vi "single_color_3D_continuous_scan_with_delay_and_ETL_control.vi"() -> ()   [LabVIEW 2017]
uses:
  <vilib>/DAQmx/write.llb/DAQmx Write (Analog DBL 1Chan 1Samp).vi
  <vilib>/DAQmx/write.llb/DAQmx Write (Analog 1D DBL NChan 1Samp).vi
  <vilib>/DAQmx/write.llb/DAQmx Write (Analog 2D DBL NChan NSamp).vi
  <vilib>/DAQmx/create/channels.llb/DAQmx Create Channel (AO-Voltage-Basic).vi
  <vilib>/DAQmx/miscellaneous.llb/DAQmx Fill In Error Info.vi
  <vilib>/Utility/file.llb/Read Delimited Spreadsheet (DBL).vi
  <vilib>/measure/mascope.llb/Transition Measurements 1 chan.vi
  <vilib>/DAQmx/configure/timing.llb/DAQmx Timing (Sample Clock).vi
  <vilib>/DAQmx/configure/trigger.llb/DAQmx Start Trigger (Digital Edge).vi
  <vilib>/DAQmx/configure/trigger.llb/DAQmx Start Trigger (None).vi
  <vilib>/measure/NI_MAPro.lvlib
panel:
  in  "Listbox":i32(listbox)=3
  in  "ETL3 (v)":dbl(slide) scale=-10.0..10.0
  out "mirx raw 2":dbl[](array[numeric])
  out "Delay":dbl
  out "Sampling rate":i32
  out "ETL3":waveform(dbl)(graph)
  out "mirror y":waveform(dbl)(graph)
  out "mirror x":waveform(dbl)(graph)
  out "Laser":waveform(dbl)(graph)
  out "camera":waveform(dbl)(graph)
  out "mirx transition duration":dbl
  out "etl3 timing array":dbl[](array[numeric])
  out "mirror y timing array":dbl[](array[numeric])
  out "mirror x timing array":dbl[](array[numeric])
  out "Laser timing array":dbl[](array[numeric])
  out "camera timing array":dbl[](array[numeric])
  out "etl raw":dbl[](array[numeric])
  out "miry raw":dbl[](array[numeric])
  out "mirx raw":dbl[](array[numeric])
  out "Laser Intensity":dbl
  out "Off Time":dbl
  out "On Time":dbl
  out "Number of slices":dbl
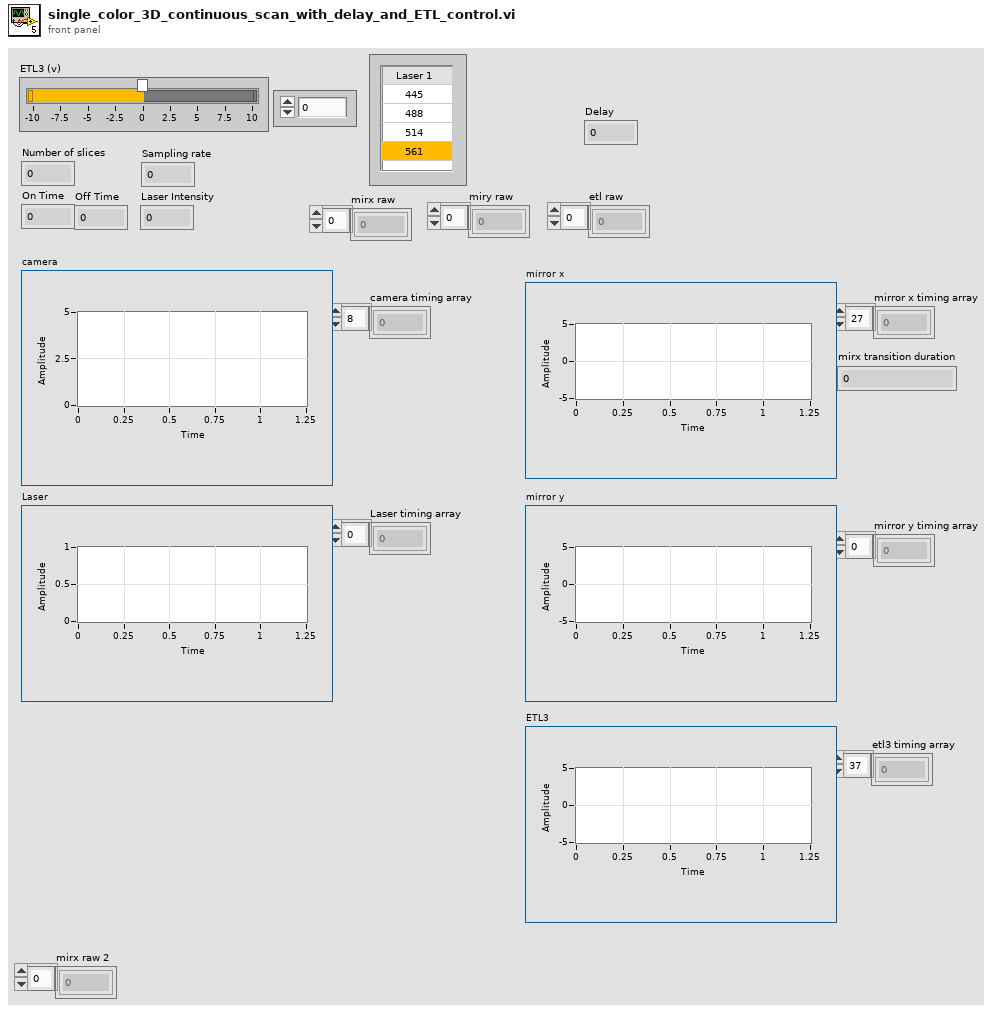
[diagram p1: front panel]
types:
  T1 = enum32{"Invalid", "Standard", "Closed", "Hidden", "Minimized", "Maximized"}
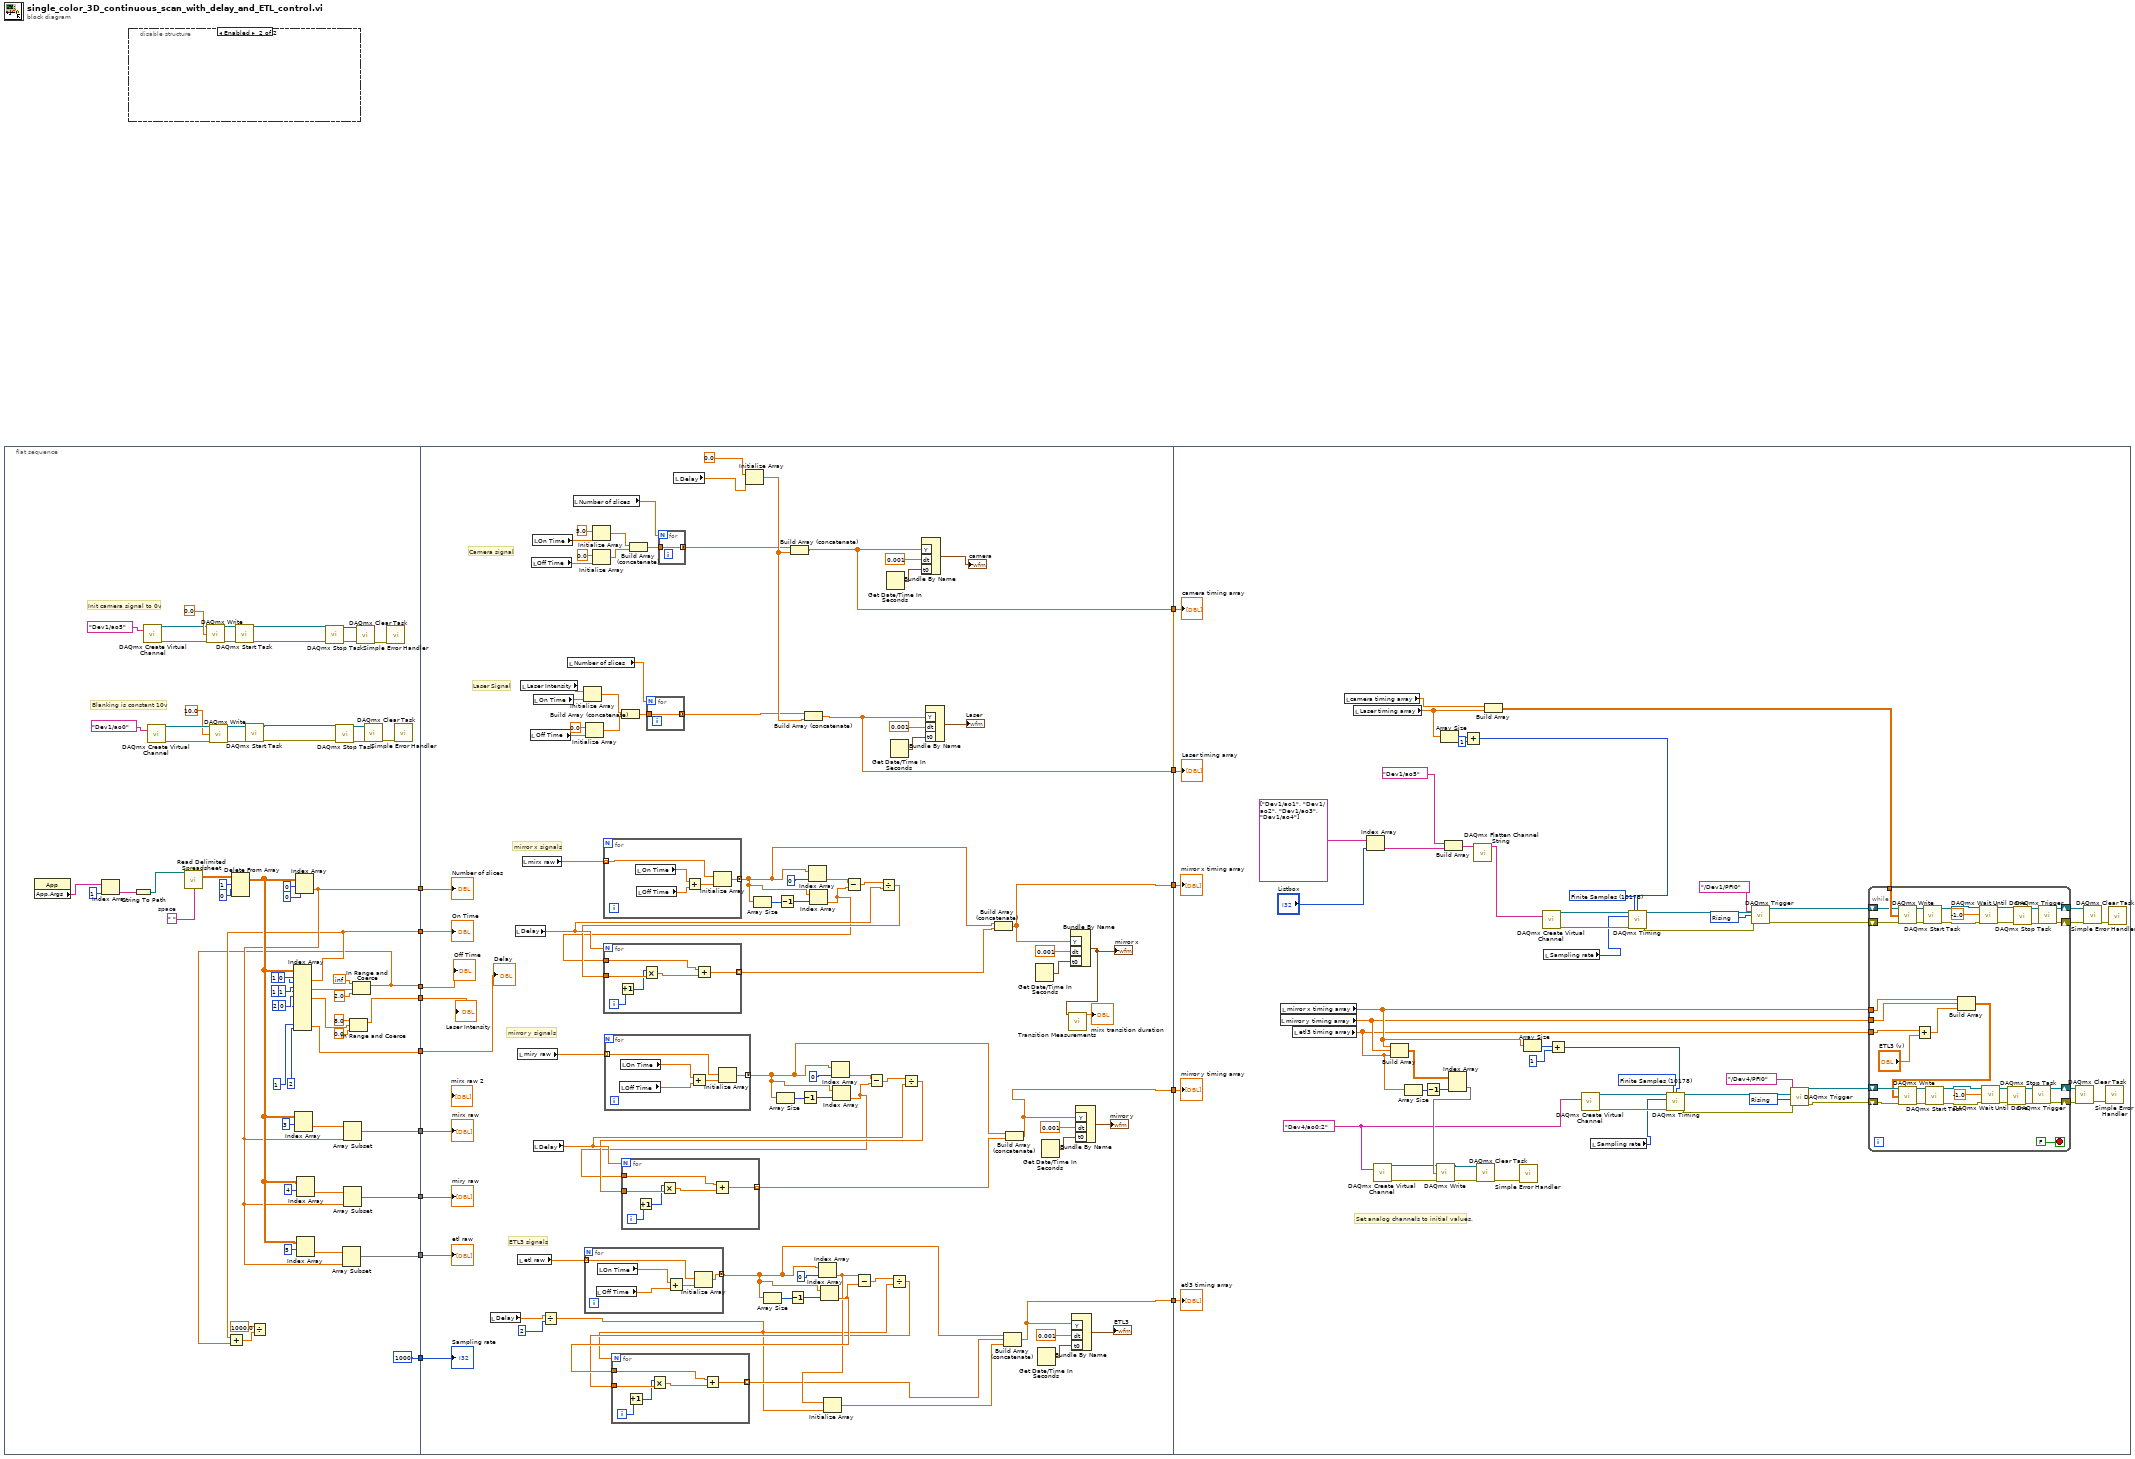
[diagram p0: block diagram]
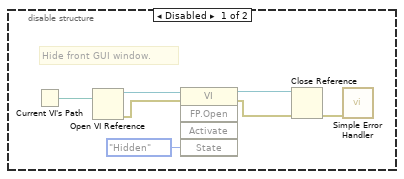
[diagram p2: hidden frame]
diagram:
  n1 = flat-sequence {
    tunnel: [w56] -> w14
    tunnel: [w42] -> w13
    tunnel: [w41] -> w12
    tunnel: [w35] -> w11
    tunnel: [w55] -> w10
    tunnel: [w54] -> w9
    tunnel: [w53] -> w8
    tunnel: [1000] -> w2
    tunnel: [w32] -> w1
    tunnel: w14 -> [w138]
    tunnel: w13 -> [w137]
    tunnel: w12 -> [w136]
    tunnel: w11 -> [w135]
    tunnel: w10 -> [w134]
    tunnel: w9 -> [w133]
    tunnel: w8 -> [w132]
    tunnel: [w131] -> w7
    tunnel: [w130] -> w6
    tunnel: [w129] -> w5
    tunnel: [w121] -> w4
    tunnel: [w120] -> w3
    tunnel: w2 -> [w122]
    tunnel: w1 -> [w118]
    tunnel: w7 -> [w231]
    tunnel: w6 -> [w230]
    tunnel: w5 -> [w229]
    tunnel: w4 -> [w228]
    tunnel: w3 -> [w227]
    frame #0 {
      w57 = " "  # space
      # "Init camera signal to 0v"
      # "Blanking is constant 10v"
      n2 = property class="App"() -> ("App.Args"=w45:string[])  [unwired: 2 in, 2 out]
      n3 = Index Array(array=w45, index=1) -> (element=w44:string)
      n4 = String To Path(string=w44) -> (path=w43:path)
      n5 = call-poly <vilib>:"DAQmx Create Virtual Channel.vi"("physical channels"=tag "Dev1/ao5") -> ("task out"=w18:refnum<k21>, "error out"=w17:errorcluster)  [unwired: 13 in]
      n6 = call-poly <vilib>:"DAQmx Create Virtual Channel.vi"("physical channels"=tag "Dev1/ao0") -> ("task out"=w51:refnum<k21>, "error out"=w52:errorcluster)  [unwired: 13 in]
      n7 = call-poly <vilib>:"Read Delimited Spreadsheet.vi"("file path (dialog if empty)"=w43, "delimiter (\\t)"=w57) -> ("all rows"=w73:dbl[][])  [unwired: 8 in, 5 out]
      n8 = call-poly <vilib>:"DAQmx Write.vi"("task/channels in"=w18, "data"=0.0, "error in"=w17) -> ("task out"=w25:refnum<k21>, "error out"=w24:errorcluster)  [unwired: 10 in, 1 out]
      n9 = call-poly <vilib>:"DAQmx Write.vi"("task/channels in"=w51, "data"=10.0, "error in"=w52) -> ("task out"=w31:refnum<k21>, "error out"=w30:errorcluster)  [unwired: 10 in, 1 out]
      n10 = Delete From Array(array=w73, length=1, index (row)=0) -> (array with subset deleted=w74:dbl[][])  [unwired: 1 in, 1 out]
      n11 = call <vilib>:"DAQmx Start Task.vi"("task/channels in"=w25, "error in"=w24) -> ("task out"=w16:refnum<k21>, "error out"=w15:errorcluster)  [unwired: 12 in]
      n12 = call <vilib>:"DAQmx Start Task.vi"("task/channels in"=w31, "error in"=w30) -> ("task out"=w27:refnum<k21>, "error out"=w26:errorcluster)  [unwired: 12 in]
      n13 = Index Array(array=w74, index (row) #1=1 ("index (row)"), index (col) #1=0 ("disabled index (col)"), index (row) #2=1 ("index (row)"), index (col) #2=1 ("disabled index (col)"), index (row) #3=2 ("index (row)"), index (col) #3=0 ("disabled index (col)"), index (row) #6=1 ("index (row)"), index (col) #6=2 ("disabled index (col)")) -> (element #1=w42:dbl, element #2=w78:dbl, element #3=w36:dbl, element #6=w32:dbl)  [unwired: 4 in, 2 out]
      n14 = Index Array(array=w74, index (row)=3) -> (element=w75:dbl[])  [unwired: 1 in]
      n15 = Index Array(array=w74, index (row)=0, index (col)=0 ("disabled index (col)")) -> (element=w56:dbl)
      n16 = Index Array(array=w74, index (row)=5) -> (element=w77:dbl[])  [unwired: 1 in]
      n17 = Index Array(array=w74, index (row)=4) -> (element=w76:dbl[])  [unwired: 1 in]
      n18 = call <vilib>:"DAQmx Stop Task.vi"("task/channels in"=w16, "error in"=w15) -> ("task out"=w22:refnum<k21>, "error out"=w23:errorcluster)  [unwired: 12 in]
      n19 = call <vilib>:"DAQmx Stop Task.vi"("task/channels in"=w27, "error in"=w26) -> ("task out"=w29:refnum<k21>, "error out"=w28:errorcluster)  [unwired: 12 in]
      n20 = Array Subset(array=w77, length=w56) -> (w53:dbl[])  [unwired: 1 in]
      n21 = Array Subset(array=w75, length=w56) -> (w55:dbl[])  [unwired: 1 in]
      n22 = Array Subset(array=w76, length=w56) -> (w54:dbl[])  [unwired: 1 in]
      n23 = In Range and Coerce(upper limit=8.0, x=w36, lower limit=0.0) -> (coerced(x)=w35:dbl)  [unwired: 1 out]
      n24 = In Range and Coerce(upper limit=inf, x=w78, lower limit=2.0) -> (coerced(x)=w41:dbl)  [unwired: 1 out]
      n25 = Add(x=w42, y=w41) -> (x+y=w39:dbl)
      n26 = Divide(x=1000.0, y=w39) -> ()  [unwired: 1 out]
      n27 = call <vilib>:"DAQmx Clear Task.vi"("task in"=w22, "error in"=w23) -> ("error out"=w19:errorcluster)  [unwired: 13 in]
      n28 = call <vilib>:"DAQmx Clear Task.vi"("task in"=w29, "error in"=w28) -> ("error out"=w50:errorcluster)  [unwired: 13 in]
      n29 = call <vilib>:"Simple Error Handler.vi"("error in (no error)"=w19) -> ()  [unwired: 4 in, 5 out]
      n30 = call <vilib>:"Simple Error Handler.vi"("error in (no error)"=w50) -> ()  [unwired: 4 in, 5 out]
    }
    frame #1 {
      # "ETL3 signals"
      # "mirror y signals"
      # "mirror x signals"
      # "Laser Signal"
      # "Camera signal"
      n31 = local read "Delay"() -> (w88:dbl)
      n32 = local read "Delay"() -> (w109:dbl)
      n33 = local read "miry raw"() -> (w150:dbl[])
      n34 = local read "etl raw"() -> (w149:dbl[])
      n35 = local read "Laser Intensity"() -> (w158:dbl)
      n36 = local read "mirx raw"() -> (w151:dbl[])
      n37 = local read "Off Time"() -> (w81:dbl)
      n38 = local read "Off Time"() -> (w163:dbl)
      n39 = local read "On Time"() -> (w164:dbl)
      n40 = local read "On Time"() -> (w157:dbl)
      n41 = local read "Delay"() -> (w99:dbl)
      n42 = Divide(x=w88, y=2 ("index")) -> (x/y=w83:dbl)
      n43 = local read "Number of slices"() -> (w153:dbl)
      n44 = local read "Number of slices"() -> (w82:dbl)
      n45 = Initialize Array(w158, w157) -> (w156:dbl[])
      n46 = for {
        tunnel: w149 -> [w181] mode=indexing
        tunnel: [w180] -> w91 mode=concatenating
        n47 = local read "Off Time"() -> (w178:dbl)
        n48 = local read "On Time"() -> (w179:dbl)
        n49 = Add(x=w179, y=w178) -> (x+y=w182:dbl)
        n50 = Initialize Array(w181, w182) -> (w180:dbl[])
      }
      n51 = Initialize Array(0.0 ("element"), w81) -> (w154:dbl[])
      n52 = Initialize Array(5.0 ("element"), w164) -> (w161:dbl[])
      n53 = Initialize Array(0.0 ("element"), w163) -> (w160:dbl[])
      n54 = for {
        tunnel: w151 -> [w197] mode=indexing
        tunnel: [w196] -> w112 mode=concatenating
        n55 = local read "On Time"() -> (w195:dbl)
        n56 = local read "Off Time"() -> (w194:dbl)
        n57 = Add(x=w195, y=w194) -> (x+y=w198:dbl)
        n58 = Initialize Array(w197, w198) -> (w196:dbl[])
      }
      n59 = for {
        tunnel: w150 -> [w186] mode=indexing
        tunnel: [w185] -> w100 mode=concatenating
        n60 = local read "Off Time"() -> (w183:dbl)
        n61 = local read "On Time"() -> (w184:dbl)
        n62 = Add(x=w184, y=w183) -> (x+y=w187:dbl)
        n63 = Initialize Array(w186, w187) -> (w185:dbl[])
      }
      n64 = Build Array (concatenate)(w156, w154) -> (w152:dbl[])
      n65 = Build Array (concatenate)(w161, w160) -> (w159:dbl[])
      n66 = for {
        N: w153 -> [_]
        tunnel: w152 -> [w199]
        tunnel: [w199] -> w79 mode=concatenating
      }
      n67 = for {
        N: w82 -> [_]
        tunnel: w159 -> [w200]
        tunnel: [w200] -> w80 mode=concatenating
      }
      n68 = local read "Delay"() -> (w117:dbl)
      n69 = Initialize Array(0.0 ("y"), w117) -> (w116:dbl[])
      n70 = Array Size(array=w112) -> (size(s)=w113:i32)
      n71 = Array Size(array=w91) -> (size(s)=w94:i32)
      n72 = Array Size(array=w100) -> (size(s)=w103:i32)
      n73 = Decrement(x=w113) -> (x-1=w111:i32)
      n74 = Decrement(x=w94) -> (x-1=w93:i32)
      n75 = Build Array (concatenate)(w80, w116) -> (w131:dbl[])
      n76 = Decrement(x=w103) -> (x-1=w102:i32)
      n77 = Build Array (concatenate)(w79, w116) -> (w130:dbl[])
      n78 = Index Array(array=w112, index=0) -> (element=w114:dbl)
      n79 = Index Array(array=w112, index=w111) -> (element=w107:dbl)
      n80 = Index Array(array=w91, index=0) -> (element=w87:dbl)
      n81 = Index Array(array=w91, index=w93) -> (element=w90:dbl)
      n82 = Initialize Array(w87, w83) -> (w84:dbl[])
      n83 = Index Array(array=w100, index=0) -> (element=w104:dbl)
      n84 = Index Array(array=w100, index=w102) -> (element=w97:dbl)
      n85 = Subtract(x=w114, y=w107) -> (x-y=w110:dbl)
      n86 = Subtract(x=w87, y=w90) -> (x-y=w92:dbl)
      n87 = Subtract(x=w104, y=w97) -> (x-y=w101:dbl)
      n88 = Divide(x=w110, y=w109) -> (x/y=w108:dbl)
      n89 = for {
        N: w109 -> [_]
        tunnel: w108 -> [w193]
        tunnel: w107 -> [w190]
        tunnel: [w188] -> w106 mode=indexing
        i -> [w192]
        n90 = Increment(x=w192) -> (x+1=w191:i32)
        n91 = Multiply(x=w191, y=w193) -> (x*y=w189:dbl)
        n92 = Add(x=w190, y=w189) -> (x+y=w188:dbl)
      }
      n93 = Get Date/Time In Seconds() -> (seconds since 1Jan1904=w145:timestamp)
      n94 = Get Date/Time In Seconds() -> (seconds since 1Jan1904=w143:timestamp)
      n95 = Divide(x=w92, y=w83) -> (x/y=w86:dbl)
      n96 = for {
        N: w83 -> [_]
        tunnel: w86 -> [w171]
        tunnel: w90 -> [w168]
        tunnel: [w166] -> w85 mode=indexing
        i -> [w170]
        n97 = Increment(x=w170) -> (x+1=w169:i32)
        n98 = Multiply(x=w169, y=w171) -> (x*y=w167:dbl)
        n99 = Add(x=w168, y=w167) -> (x+y=w166:dbl)
      }
      n100 = Divide(x=w101, y=w99) -> (x/y=w98:dbl)
      n101 = for {
        N: w99 -> [_]
        tunnel: w98 -> [w177]
        tunnel: w97 -> [w174]
        tunnel: [w172] -> w96 mode=indexing
        i -> [w176]
        n102 = Increment(x=w176) -> (x+1=w175:i32)
        n103 = Multiply(x=w175, y=w177) -> (x*y=w173:dbl)
        n104 = Add(x=w174, y=w173) -> (x+y=w172:dbl)
      }
      n105 = Bundle By Name("Y"=w131, "dt"=0.001, "t0"=w145) -> (→"camera":waveform(dbl))  [unwired: 1 in]
      n106 = Bundle By Name("Y"=w130, "dt"=0.001, "t0"=w143) -> (→"Laser":waveform(dbl))  [unwired: 1 in]
      n107 = Build Array (concatenate)(w112, w106) -> (w129:dbl[])
      n108 = Build Array (concatenate)(w91, w85, w84) -> (w120:dbl[])
      n109 = Build Array (concatenate)(w100, w96) -> (w121:dbl[])
      n110 = Get Date/Time In Seconds() -> (seconds since 1Jan1904=w147:timestamp)
      n111 = Get Date/Time In Seconds() -> (seconds since 1Jan1904=w139:timestamp)
      n112 = Get Date/Time In Seconds() -> (seconds since 1Jan1904=w141:timestamp)
      n113 = Bundle By Name("Y"=w129, "dt"=0.001, "t0"=w147) -> (w125:waveform(dbl))  [unwired: 1 in]
      "mirror x" <- w125
      n114 = call-poly <vilib>:"Transition Measurements.vi"("signal in"=w125) -> ("transition duration"=→"mirx transition duration":dbl)  [unwired: 5 in, 5 out]
      n115 = Bundle By Name("Y"=w120, "dt"=0.001, "t0"=w139) -> (→"ETL3":waveform(dbl))  [unwired: 1 in]
      n116 = Bundle By Name("Y"=w121, "dt"=0.001, "t0"=w141) -> (→"mirror y":waveform(dbl))  [unwired: 1 in]
      "Number of slices" <- w138
      "On Time" <- w137
      "Off Time" <- w136
      "Laser Intensity" <- w135
      "mirx raw" <- w134
      "miry raw" <- w133
      "etl raw" <- w132
      "Sampling rate" <- w122
      "Delay" <- w118
    }
    frame #2 {
      w237 = 10280 items=["Rising"=10280, "Falling"=10171] ("edge")
      w235 = 10178 items=["Finite Samples"=10178, "Continuous Samples"=10123, "Hardware Timed Single Point"=12522] ("sample mode")
      w236 = tag "Dev4/ao0:2" ("physical channels")
      w233 = 10280 items=["Rising"=10280, "Falling"=10171] ("edge")
      w232 = 10178 items=["Finite Samples"=10178, "Continuous Samples"=10123, "Hardware Timed Single Point"=12522] ("sample mode")
      # "Set analog channels to initial values."
      n117 = local read "mirror y timing array"() -> (w209:dbl[])
      n118 = local read "mirror x timing array"() -> (w210:dbl[])
      n119 = local read "etl3 timing array"() -> (w208:dbl[])
      n120 = local read "camera timing array"() -> (w248:dbl[])
      n121 = local read "Laser timing array"() -> (w201:dbl[])
      n122 = Index Array(array=tag[] ["Dev1/ao1", "Dev1/ao2", "Dev1/ao3", "Dev1/ao4"], index="Listbox") -> (element=w203:tag)
      n123 = call-poly <vilib>:"DAQmx Create Virtual Channel.vi"("physical channels"=w236) -> ("task out"=w244:refnum<k21>, "error out"=w245:errorcluster)  [unwired: 13 in]
      n124 = Build Array(w210, w209, w208) -> (w258:dbl[][])
      n125 = Array Size(array=w208) -> (size(s)=w250:i32)
      n126 = Decrement(x=w250) -> (x-1=w251:i32)
      n127 = Array Size(array=w201) -> (size(s)=w217:i32)
      n128 = Build Array(tag "Dev1/ao5" ("physical channels"), w203) -> (w205:tag[])
      n129 = Index Array(array=w258, index (col)=w251) -> (element=w252:dbl[])  [unwired: 1 in]
      n130 = call-poly <vilib>:"DAQmx Write.vi"("task/channels in"=w244, "data"=w252, "error in"=w245) -> ("task out"=w246:refnum<k21>, "error out"=w247:errorcluster)  [unwired: 10 in, 1 out]
      n131 = Add(x=w217, y=1) -> (x+y=w215:i32)
      n132 = call <vilib>:"DAQmx Flatten Channel String.vi"("names in"=w205) -> ("names out"=w202:string)  [unwired: 13 in, 1 out]
      n133 = call <vilib>:"DAQmx Clear Task.vi"("task in"=w246, "error in"=w247) -> ("error out"=w259:errorcluster)  [unwired: 13 in]
      n134 = Build Array(w248, w201) -> (w249:dbl[][])
      n135 = call <vilib>:"Simple Error Handler.vi"("error in (no error)"=w259) -> ()  [unwired: 4 in, 5 out]
      n136 = Array Size(array=w210) -> (size(s)=w220:i32)
      n137 = call-poly <vilib>:"DAQmx Create Virtual Channel.vi"("physical channels"=w202) -> ("task out"=w240:refnum<k21>, "error out"=w241:errorcluster)  [unwired: 13 in]
      n138 = local read "Sampling rate"() -> (w226:i32)
      n139 = Add(x=w220, y=1) -> (x+y=w218:i32)
      n140 = call-poly <vilib>:"DAQmx Create Virtual Channel.vi"("physical channels"=w236) -> ("task out"=w254:refnum<k21>, "error out"=w255:errorcluster)  [unwired: 13 in]
      n141 = local read "Sampling rate"() -> (w225:i32)
      n142 = call-poly <vilib>:"DAQmx Timing.vi"("task/channels in"=w240, "sample mode"=w232, "samples per channel"=w215, "rate"=w226, "error in"=w241) -> ("task out"=w242:refnum<k21>, "error out"=w243:errorcluster)  [unwired: 9 in]
      n143 = call-poly <vilib>:"DAQmx Timing.vi"("task/channels in"=w254, "sample mode"=w235, "samples per channel"=w218, "rate"=w225, "error in"=w255) -> ("task out"=w256:refnum<k21>, "error out"=w257:errorcluster)  [unwired: 9 in]
      n144 = call-poly <vilib>:"DAQmx Trigger.vi"("task/channels in"=w242, "source"=tag "/Dev1/PFI0", "edge"=w233, "error in"=w243) -> ("task out"=w224:refnum<k21>, "error out"=w223:errorcluster)  [unwired: 10 in]
      n145 = call-poly <vilib>:"DAQmx Trigger.vi"("task/channels in"=w256, "source"=tag "/Dev4/PFI0", "edge"=w237, "error in"=w257) -> ("task out"=w222:refnum<k21>, "error out"=w221:errorcluster)  [unwired: 10 in]
      n146 = while {
        tunnel: w249 -> [w289]
        shift-right: [w268] -> w212
        shift-left: w224 -> [w282]
        shift-right: [w267] -> w211
        shift-left: w223 -> [w281]
        shift-right: [w274] -> w214
        shift-left: w222 -> [w280]
        shift-right: [w273] -> w213
        shift-left: w221 -> [w279]
        tunnel: w210 -> [w264]
        tunnel: w209 -> [w263]
        tunnel: w208 -> [w262]
        stop <- FALSE stop-if-true
        n147 = call-poly <vilib>:"DAQmx Write.vi"("task/channels in"=w282, "data"=w289, "error in"=w281) -> ("task out"=w287:refnum<k21>, "error out"=w288:errorcluster)  [unwired: 10 in, 1 out]
        n148 = Add(x=w262, y="ETL3 (v)") -> (x+y=w260:dbl[])
        n149 = call <vilib>:"DAQmx Start Task.vi"("task/channels in"=w287, "error in"=w288) -> ("task out"=w286:refnum<k21>, "error out"=w285:errorcluster)  [unwired: 12 in]
        n150 = Build Array(w264, w263, w260) -> (w266:dbl[][])
        n151 = call-poly <vilib>:"DAQmx Write.vi"("task/channels in"=w280, "data"=w266, "error in"=w279) -> ("task out"=w292:refnum<k21>, "error out"=w293:errorcluster)  [unwired: 10 in, 1 out]
        n152 = call <vilib>:"DAQmx Start Task.vi"("task/channels in"=w292, "error in"=w293) -> ("task out"=w291:refnum<k21>, "error out"=w290:errorcluster)  [unwired: 12 in]
        n153 = call <vilib>:"DAQmx Wait Until Done.vi"("task/channels in"=w286, "timeout (sec)"=-1.0, "error in"=w285) -> ("task out"=w270:refnum<k21>, "error out"=w269:errorcluster)  [unwired: 11 in]
        n154 = call <vilib>:"DAQmx Wait Until Done.vi"("task/channels in"=w291, "timeout (sec)"=-1.0, "error in"=w290) -> ("task out"=w278:refnum<k21>, "error out"=w277:errorcluster)  [unwired: 11 in]
        n155 = call <vilib>:"DAQmx Stop Task.vi"("task/channels in"=w278, "error in"=w277) -> ("task out"=w276:refnum<k21>, "error out"=w275:errorcluster)  [unwired: 12 in]
        n156 = call <vilib>:"DAQmx Stop Task.vi"("task/channels in"=w270, "error in"=w269) -> ("task out"=w272:refnum<k21>, "error out"=w271:errorcluster)  [unwired: 12 in]
        n157 = call-poly <vilib>:"DAQmx Trigger.vi"("task/channels in"=w276, "error in"=w275) -> ("task out"=w274:refnum<k21>, "error out"=w273:errorcluster)  [unwired: 12 in]
        n158 = call-poly <vilib>:"DAQmx Trigger.vi"("task/channels in"=w272, "error in"=w271) -> ("task out"=w268:refnum<k21>, "error out"=w267:errorcluster)  [unwired: 12 in]
      }
      n159 = call <vilib>:"DAQmx Clear Task.vi"("task in"=w214, "error in"=w213) -> ("error out"=w253:errorcluster)  [unwired: 13 in]
      n160 = call <vilib>:"DAQmx Clear Task.vi"("task in"=w212, "error in"=w211) -> ("error out"=w239:errorcluster)  [unwired: 13 in]
      n161 = call <vilib>:"Simple Error Handler.vi"("error in (no error)"=w253) -> ()  [unwired: 4 in, 5 out]
      n162 = call <vilib>:"Simple Error Handler.vi"("error in (no error)"=w239) -> ()  [unwired: 4 in, 5 out]
      "camera timing array" <- w231
      "Laser timing array" <- w230
      "mirror x timing array" <- w229
      "mirror y timing array" <- w228
      "etl3 timing array" <- w227
    }
  }
  n163 = disable-structure shown="Enabled" {
    frame Disabled {
      # "Hide front GUI window."
      n164 = Current VI's Path() -> (path=w300:path)
      n165 = Open VI Reference(vi path=w300) -> (vi reference=w298:refnum<vi>, error out=w297:errorcluster)  [unwired: 5 in]
      n166 = invoke class="VI" method="FP.Open"(reference=w298, error in=w297, "State"=T1."Hidden") -> (reference out=w296:refnum<vi>, error out=w295:errorcluster)  [unwired: 2 in, 3 out]
      n167 = Close Reference(reference=w296, error in (no error)=w295) -> (error out=w299:errorcluster)
      n168 = call <vilib>:"Simple Error Handler.vi"("error in (no error)"=w299) -> ()  [unwired: 4 in, 5 out]
    }
    frame Enabled {
    }
  }
